vi "Launch GoBang Server.vi"() -> ()   [LabVIEW 2014, in "GoBang.lvlib"]
uses:
  GoBang.lvlib
  CS++GoBangServer.lvclass
  <vilib>/ActorFramework/Message Enqueuer/Message Enqueuer.lvclass/Message Enqueuer.ctl
  <vilib>/ActorFramework/Message Enqueuer/Enqueue.vi
  <vilib>/ActorFramework/Message Priority Queue/Priority Enqueue.vi
  <vilib>/ActorFramework/Stop Msg/Stop Msg.lvclass
  <vilib>/ActorFramework/Actor/Actor.lvclass
panel:
  in  "Stop":bool
  out "error out":errorcluster
  in  "Open FP":bool
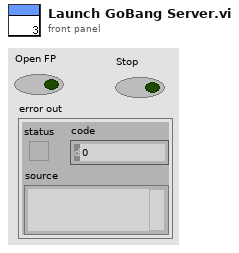
[diagram p1: front panel]
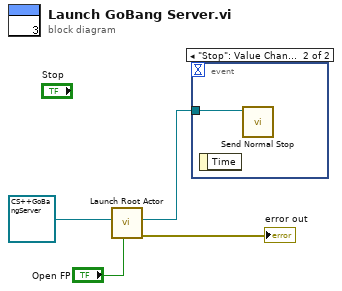
[diagram p0: block diagram]
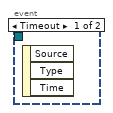
[diagram p2: hidden frame]
diagram:
  n1 = call <vilib>:"Launch Root Actor.vi"("Open Actor Core front panel? (F)"="Open FP", "Actor"=refnum<class "CS++GoBangServer.lvclass"> refnum ("GoBang.lvlib:CS++GoBangServer.lvclass")) -> ("error out"=→"error out":errorcluster, "Actor's Enqueuer"=w1:refnum<class "Message Enqueuer.lvclass">)  [unwired: 8 in]
  n2 = event shown="[1] \"Stop\": Value Change" {
    selector: _ -> [_ _]
    dyn-events: _ -> [_ _]
    timeout: _ -> [_ _]
    tunnel: w1 -> [_ w5]
    event Timeout {
      n3 = event-data() -> ()  [unwired: 1 in, 3 out]
    }
    event "Stop": Value Change {
      n4 = event-data() -> ()  [unwired: 1 in, 1 out]
      n5 = call <vilib>:"Send Normal Stop.vi"("Message Enqueuer"=w5) -> ()  [unwired: 10 in, 1 out]
    }
  }
